vi "Thread Parameters.Set Processor.vi"(10 "Processor":i32=-2, 11 "Thread Parameters in":refnum<class "Thread Parameters.lvclass">) -> (3 "Thread Parameters out":refnum<class "Thread Parameters.lvclass">)   [LabVIEW 2017, in "DSF.Engine.lvlib" / "Thread Parameters.lvclass"]
uses:
  Thread Parameters.lvclass
  Thread Parameters.lvclass/Thread Parameters.ctl
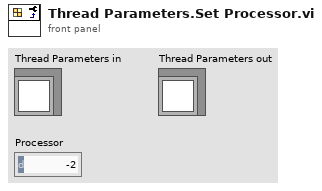
[diagram p1: front panel]
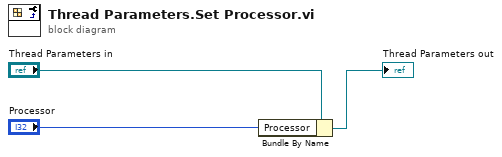
[diagram p0: block diagram]
diagram:
  n1 = Bundle By Name(cluster="Thread Parameters in", "Processor"="Processor") -> (→"Thread Parameters out":refnum<class "Thread Parameters.lvclass">)
